vi "Std Atm.vi"(4 "O2%":dbl=15.0, 6 "Pressure Pa":dbl=84307.3, 7 "Air pressure Pa":dbl=84307.3, 8 "Alt M":dbl=1524.0) -> (1 "Alt Eff M":dbl=4156.670008894815, 2 "Alt M":dbl=1523.996203731578, 3 "Air pressure Pa":dbl=84307.26094236002)   [LabVIEW 2012]
panel:
  out "Ratio":dbl=0.5960231799713962
  out "PO2":dbl=12646.095
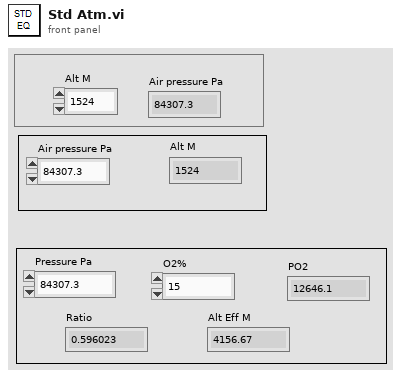
[diagram p1: front panel]
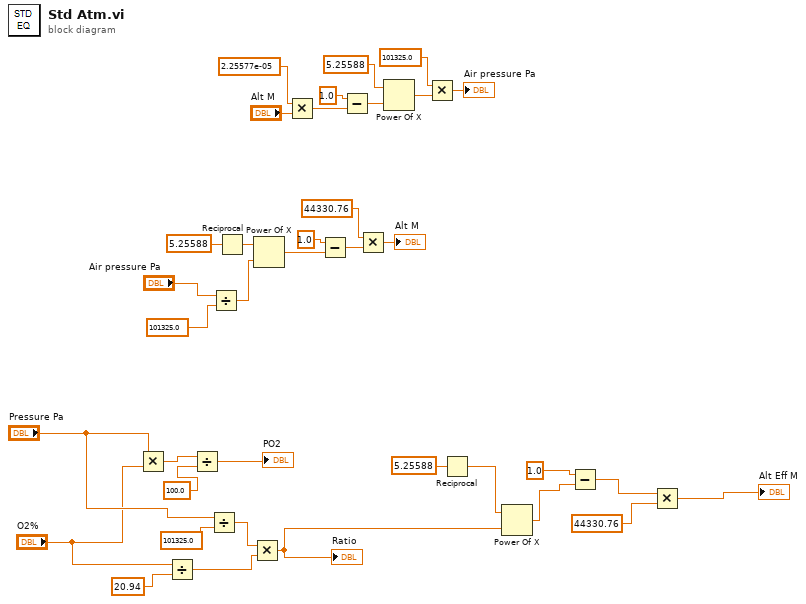
[diagram p0: block diagram]
diagram:
  n1 = Multiply(x="Pressure Pa", y="O2%") -> (x*y=w17:dbl)
  n2 = Divide(x="O2%", y=20.94) -> (x/y=w12:dbl)
  n3 = Divide(x=w17, y=100.0 ("x")) -> (x/y=→"PO2":dbl)
  n4 = Divide(x="Pressure Pa", y=101325.0) -> (x/y=w11:dbl)
  n5 = Divide(x="Air pressure Pa", y=101325.0) -> (x/y=w22:dbl)
  n6 = Reciprocal(x=5.25588 ("y")) -> (1/x=w20:dbl)
  n7 = Multiply(x=w11, y=w12) -> (x*y=w8:dbl)
  "Ratio" <- w8
  n8 = Power Of X(1:w22, 2:w20) -> (0:w19:dbl)
  n9 = Multiply(x=2.25577e-05, y="Alt M") -> (x*y=w33:dbl)
  n10 = Subtract(x=1.0 ("y"), y=w19) -> (x-y=w18:dbl)
  n11 = Subtract(x=1.0 ("y"), y=w33) -> (x-y=w32:dbl)
  n12 = Multiply(x=44330.76, y=w18) -> (x*y=→"Alt M":dbl)
  n13 = Power Of X(1:w32, 2:5.25588 ("y")) -> (0:w30:dbl)
  n14 = Multiply(x=101325.0, y=w30) -> (x*y=→"Air pressure Pa":dbl)
  n15 = Reciprocal(x=5.25588 ("y")) -> (1/x=w1:dbl)
  n16 = Power Of X(1:w8, 2:w1) -> (0:w9:dbl)
  n17 = Subtract(x=1.0, y=w9) -> (x-y=w5:dbl)
  n18 = Multiply(x=w5, y=44330.76) -> (x*y=→"Alt Eff M":dbl)
